vi "FdxCmdEDESubControlCvi.vi"(8 "error in":errorcluster, 9 "EDESubCntlIn":T1, 10 "EDESubscriberHandle":u32, 11 "InstrumentHandle":u32) -> (0 "error out":errorcluster, 2 "EDESubscriberHandleOut":u32, 3 "InstrumentHandle":u32)   [LabVIEW 2020, in "AIM664LV.lvlib"]
doc: "This function is used to control the EDE subscriber."
uses:
  AIM664LV.lvlib
  AFDX_LibraryAdmin/FdxGlobalDllPath.vi
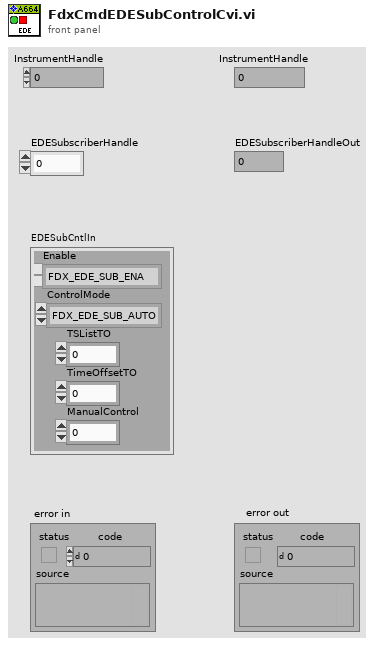
[diagram p1: front panel]
types:
  T1 = cluster{"Enable":enum32{"FDX_EDE_SUB_ENA", "FDX_EDE_SUB_DIS"}, "ControlMode":enum32{"FDX_EDE_SUB_AUTO"}, "TSListTO":u32, "TimeOffsetTO":u32, "ManualControl":u32}
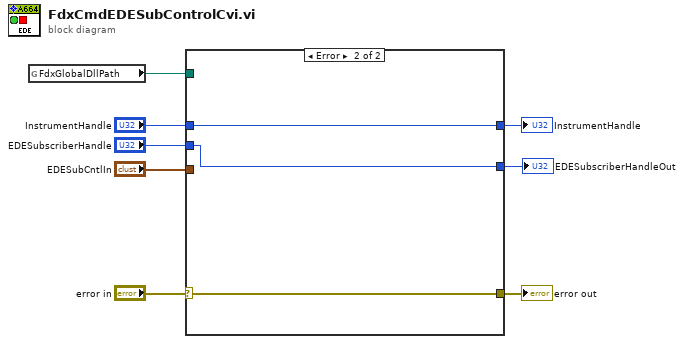
[diagram p0: block diagram]
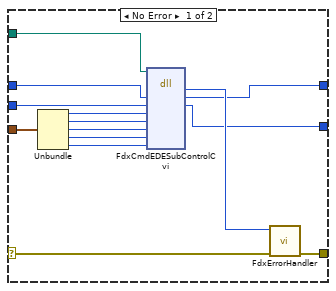
[diagram p2: hidden frame]
diagram:
  n1 = global read "FdxGlobalDllPath.vi" "FdxGlobalDllPath"() -> (w6:path)
  n2 = case shown="Error" "error in" {
    selector: "error in" -> [w21 w25]
    tunnel: [w22 w25] -> w8
    tunnel: w6 -> [w14 _]
    tunnel: [w13 w24] -> w5
    tunnel: "InstrumentHandle" -> [w12 w24]
    tunnel: "EDESubCntlIn" -> [w11 _]
    tunnel: "EDESubscriberHandle" -> [w10 w23]
    tunnel: [w9 w23] -> w1
    frame No Error {
      n3 = Unbundle(w11) -> ("Enable"=w19:enum32{"FDX_EDE_SUB_ENA", "FDX_EDE_SUB_DIS"}, "ControlMode"=w18:enum32{"FDX_EDE_SUB_AUTO"}, "TSListTO"=w17:u32, "TimeOffsetTO"=w16:u32, "ManualControl"=w15:u32)
      n4 = dll-call lib="aim_fdx.19.dll" fn="FdxCmdEDESubControlCvi"(path in=w14, "InstrumentHandle"=w12, "EDESubscriberHandle"=w10, "Enable"=w19, "ControlMode"=w18, "TSListTO"=w17, "TimeOffsetTO"=w16, "ManualControl"=w15) -> ("status"=w20:i32, "InstrumentHandle"=w13:u32, "EDESubscriberHandle"=w9:u32)  [unwired: 5 in, 4 out]
      n5 = call "FdxErrorHandler.vi"("error in"=w21, "AIM Error"=w20) -> ("error out"=w22:errorcluster)  [unwired: 9 in]
    }
    frame Error {
    }
  }
  "error out" <- w8
  "InstrumentHandle" <- w5
  "EDESubscriberHandleOut" <- w1
